vi "Change the pixel size in Tiff file metadata.vi"(8 "error in (no error)":errorcluster, 9 "Unit":u32(ring)=3 items=["None"=1, "Inch"=2, "Centimeter"=3], 10 "Pixels per unit":T1, 11 "path to TIFF file":path=path "/HD1/Users/herbertlooser/Desktop/Ladungsspr焗er.tif") -> (0 "error out":errorcluster)   [LabVIEW 2015, in "Tiff reader.lvlib"]
doc: "This .vi is taken from an online tiff reader. It is able to read 32-bit floating point .tiff images."
uses:
  Tiff reader.lvlib
panel:
  out "Progress":i32
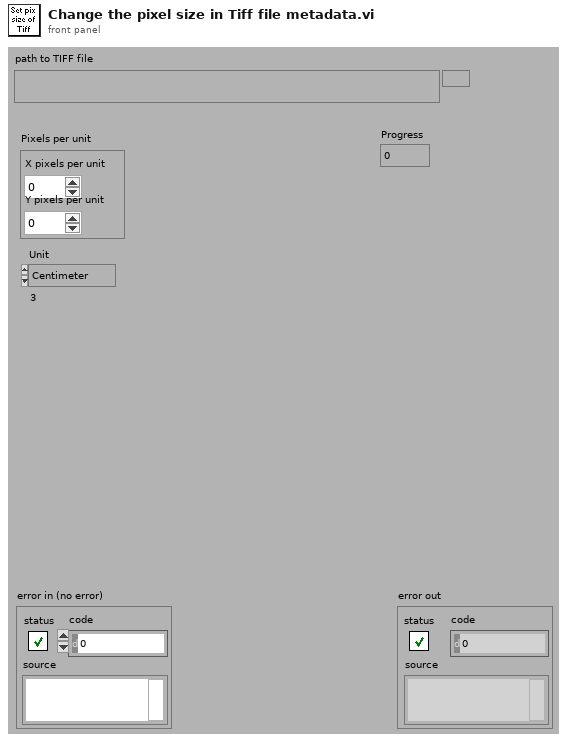
[diagram p1: front panel]
types:
  T1 = cluster{"X pixels per unit":dbl, "Y pixels per unit":dbl}
  T2 = enum16{"open", "open or create", "create or replace", "create"}
  T3 = typedef "Tiff reader.lvlib/IFD Entry.ctl" = cluster{"Tag":u16, "Type":T4, "Count":u32, "Val/Offs":u32, "Is Pointer?":bool, "Byte stream index":i32}
  T4 = typedef "Tiff reader.lvlib/FieldTypes.ctl" = enum16{"NULL", "U8", "ASCII7", "U16", "U32", "RATIONAL", "SByte(I8)", "Undef(8Bit)", "I16", "I32", "SRat(4B:4B)", "SGL(4Byte)", "DBL(8Byte)"}
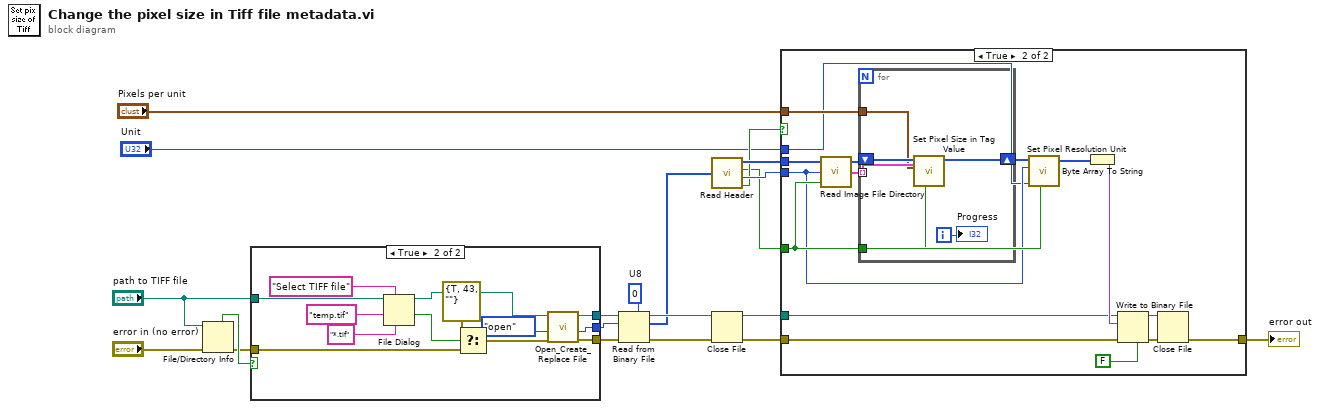
[diagram p0: block diagram]
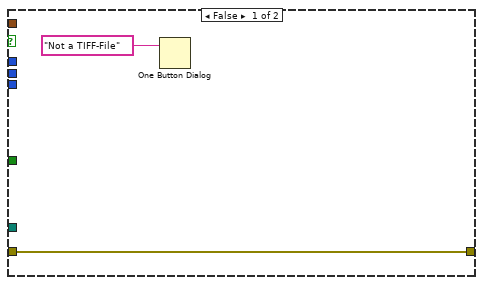
[diagram p2: hidden frame]
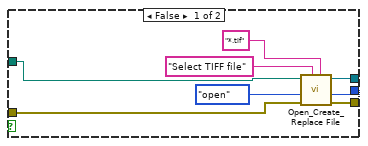
[diagram p3: hidden frame]
diagram:
  w2 = u8 0  # U8
  n1 = File/Directory Info(path="path to TIFF file", error in="error in (no error)") -> (directory=w17:bool, error out=w10:errorcluster)  [unwired: 5 out]
  n2 = case shown="True" w17 {
    tunnel: [w25 w34] -> w20
    tunnel: [w24 w36] -> w19
    tunnel: [w23 w35] -> w18
    tunnel: w10 -> [w22 w32]
    tunnel: "path to TIFF file" -> [w21 w30]
    frame False {
      n3 = call <vilib>:"Open_Create_Replace File.vi"("pattern"="*.tif", "prompt"="Select TIFF file", "error in (no error)"=w22, "function (open:0)"=T2."open", "file path"=w21) -> ("error out"=w23:errorcluster, "file size (bytes)"=w25:i32, "refnum"=w24:refnum<file>)  [unwired: 2 in, 2 out]
    }
    frame True {
      n4 = File Dialog(6:"*.tif" ("pattern"), 7:"Select TIFF file" ("prompt"), 9:"temp.tif" ("default name"), 11:w30) -> (1:w33:bool, 3:w38:path)  [unwired: 1 in, 4 out]
      n5 = Select(t=errorcluster {"status"=TRUE, "code"=43, "source"=""} ("error in (no error)"), s=w33, f=w32) -> (s? t:f=w31:errorcluster)
      n6 = call <vilib>:"Open_Create_Replace File.vi"("error in (no error)"=w31, "function (open:0)"=T2."open", "file path"=w38) -> ("error out"=w35:errorcluster, "file size (bytes)"=w34:i32, "refnum"=w36:refnum<file>)  [unwired: 3 in, 3 out]
    }
  }
  n7 = Read from Binary File(5:w2, 8:w18, 10:w20, 11:w19) -> (0:w6:errorcluster, 2:w1:u8[], 3:w7:refnum<file>)  [unwired: 3 out]
  n8 = call "Read Header.vi"("TIFF Data in"=w1) -> ("TIFF Data out"=w15:u8[], "Litt/BigEnd"=w12:bool, "ImFileDirectOffs"=w14:u32, "IsTIFF?"=w13:bool)
  n9 = Close File(refnum=w7, error in=w6) -> (path=w8:path, error out=w5:errorcluster)
  n10 = case shown="True" w13 {
    tunnel: w15 -> [_ w59]
    tunnel: w14 -> [_ w45]
    tunnel: w12 -> [_ w46]
    tunnel: w5 -> [w42 w53]
    tunnel: [w42 w50] -> w4
    tunnel: "Pixels per unit" -> [_ w56]
    tunnel: w8 -> [_ w54]
    tunnel: "Unit" -> [_ w44]
    frame False {
      n11 = One Button Dialog(message="Not a TIFF-File") -> ()  [unwired: 2 out]
    }
    frame True {
      n12 = call "Read Image File Directory.vi"("Litt/BigEnd"=w46, "Im_File_Dir Offs"=w45, "Image Data in"=w59) -> ("Directories"=w57:cluster{"Tags":T3[]}[], "Image Data out"=w58:u8[])  [unwired: 1 out]
      n13 = for {
        tunnel: w46 -> [w62]
        tunnel: w57 -> [w63] mode=indexing
        shift-right: [w61] -> w48
        shift-left: w58 -> [w64]
        tunnel: w56 -> [w60]
        i -> [w65]
        n14 = call "Set Pixel Size in Tag Value.vi"("Litt/BigEnd"=w62, "DirEntries"=w63, "Pixels per unit"=w60, "Image Data in"=w64) -> ("Image Data out"=w61:u8[])  [unwired: 4 out]
        "Progress" <- w65
      }
      n15 = call "Set Pixel Resolution Unit.vi"("Image Data in"=w48, "Im_File_Dir Offs"=w45, "Unit"=w44, "Litt/BigEnd"=w46) -> ("Image Data out"=w47:u8[])  [unwired: 3 out]
      n16 = Byte Array To String(unsigned byte array=w47) -> (string=w55:string)
      n17 = Write to Binary File(file (use dialog)=w54, data=w55, error in=w53, 5:FALSE ("prepend array or string size? (T)")) -> (refnum out=w52:refnum<file>, error out=w51:errorcluster)  [unwired: 3 out]
      n18 = Close File(refnum=w52, error in=w51) -> (error out=w50:errorcluster)  [unwired: 1 out]
    }
  }
  "error out" <- w4
